vi "SplashSreen.vi"() -> ()   [LabVIEW 2016]
panel:
  out "path":string
  out "Slide":dbl(slide) scale=0.0..10.0
  # "Body Analyser"
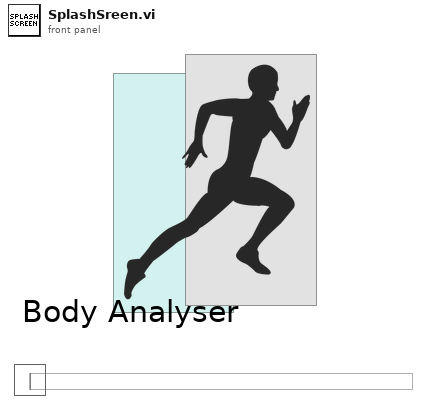
[diagram p1: front panel]
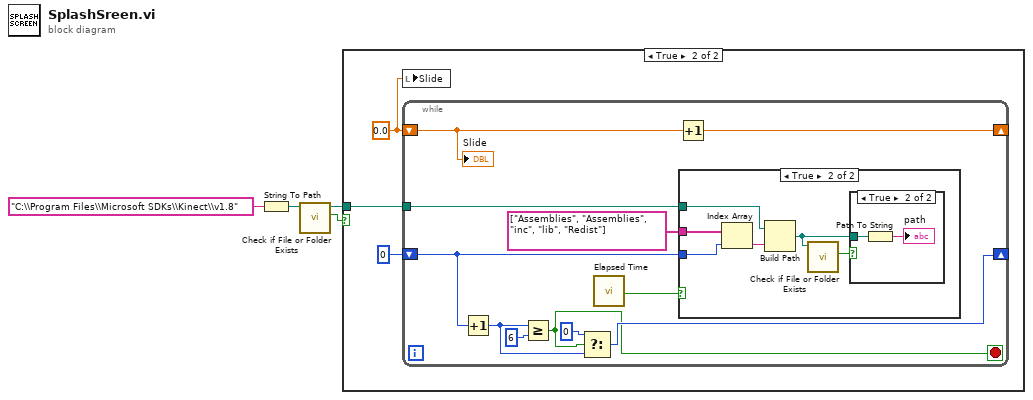
[diagram p0: block diagram]
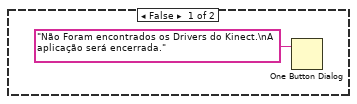
[diagram p2: hidden frame]
diagram:
  n1 = String To Path(string="C:\\Program Files\\Microsoft SDKs\\Kinect\\v1.8") -> (path=w3:path)
  n2 = call <vilib>:"Check if File or Folder Exists.vi"("path"=w3) -> ("file or folder exists?"=w1:bool, "dup path"=w2:path)  [unwired: 8 in, 1 out]
  n3 = case shown="True" w1 {
    tunnel: w2 -> [_ w6]
    frame False {
      n4 = One Button Dialog(message="Não Foram encontrados os Drivers do Kinect.\nA aplicação será encerrada.") -> ()  [unwired: 1 in, 1 out]
    }
    frame True {
      w8 = 0.0
      n5 = local write "Slide"(w8) -> ()
      n6 = while {
        shift-right: [w19] -> _
        shift-left: w8 -> [w18]
        shift-right: [w12] -> _
        shift-left: 0 -> [w16]
        tunnel: w6 -> [w10]
        stop <- w9 stop-if-true
        n7 = Increment(x=w16) -> (x+1=w13:i32)
        n8 = Greater Or Equal?(x=w13, y=6) -> (x >= y?=w9:bool)
        n9 = Select(t=0 ("y"), s=w9, f=w13) -> (s? t:f=w12:i32)
        n10 = call "Elapsed Time"() -> ("Time has Elapsed"=w17:bool)  [unwired: 12 in, 7 out]
        n11 = Increment(x=w18) -> (x+1=w19:dbl)
        n12 = case shown="True" w17 {
          tunnel: w16 -> [_ w25]
          tunnel: string[] ["Assemblies", "Assemblies", "inc", "lib", "Redist"] -> [_ w24]
          tunnel: w10 -> [_ w23]
          frame False {
          }
          frame True {
            n13 = Index Array(array=w24, index=w25) -> (element=w22:string)
            n14 = Build Path(base path=w23, name or relative path=w22) -> (appended path=w20:path)
            n15 = call <vilib>:"Check if File or Folder Exists.vi"("path"=w20) -> ("file or folder exists?"=w21:bool)  [unwired: 8 in, 2 out]
            n16 = case shown="True" w21 {
              tunnel: w20 -> [_ w27]
              frame False {
              }
              frame True {
                n17 = Path To String(path=w27) -> (string=→"path":string)
              }
            }
          }
        }
        "Slide" <- w18
      }
    }
  }
